vi "Get NextGen XML DataType For Control.vi"(8 "error in (no error)":errorcluster, 11 "Ctl Refnum":refnum<vi>) -> (0 "error out":errorcluster, 3 "String":string)   [LabVIEW 2020, in "Web Service Description.lvlib" / "NextGenXMLTypeGenerator.lvclass"]
uses:
  <vilib>/AppBuilder/Engine/WebServiceDescription/NextGenXMLTypeGenerator/NextGenXMLTypeGenerator.lvclass
  e:/builds/penguin/labview/branches/2020/dev/dist/vi.lib/AppBuilder/Engine/WebServiceDescription/LVDataTypes/LVTypeVisitor/LVTypeVisitor.lvclass
  <vilib>/AppBuilder/Engine/WebServiceDescription/LVDataTypes/LVType/LVType.lvclass
  <vilib>/AppBuilder/Engine/WebServiceDescription/LVDataTypes/LVDataTypes.lvlib
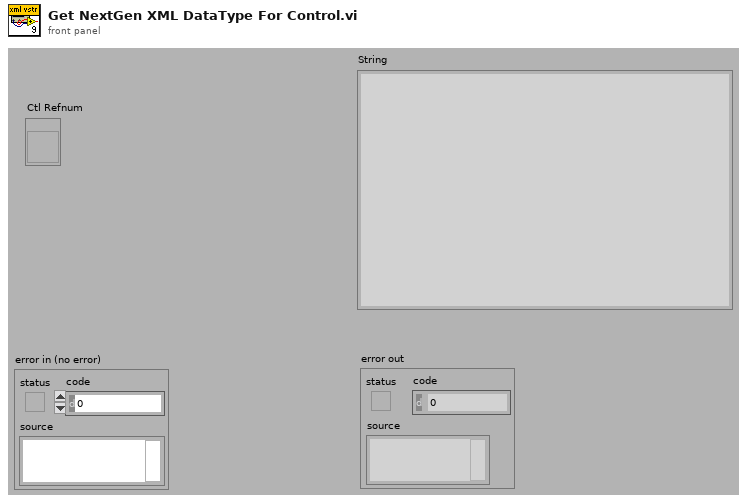
[diagram p1: front panel]
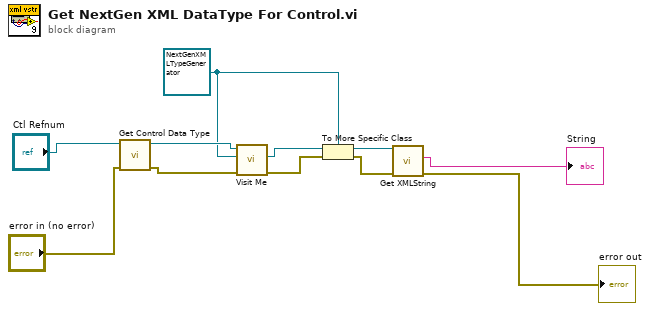
[diagram p0: block diagram]
diagram:
  w6 = refnum<class "NextGenXMLTypeGenerator.lvclass"> refnum ("NextGenXMLTypeGenerator.lvclass")
  n1 = call <vilib>:"Get Control Data Type.vi"("error in (no error)"="error in (no error)", "Ctl Refnum"="Ctl Refnum") -> ("error out"=w9:errorcluster, "Type"=w10:refnum<class "LVType.lvclass">)  [unwired: 8 out]
  n2 = call-dynamic "Visit Me.vi"("error in (no error)"=w9, "Visitor In"=w6, "LVType in"=w10) -> ("error out"=w8:errorcluster, "Visitor Out"=w7:refnum<class "LVTypeVisitor.lvclass">)  [unwired: 7 out]
  n3 = To More Specific Class(target class=w6, reference=w7, error in=w8) -> (specific class reference=w4:refnum<class "NextGenXMLTypeGenerator.lvclass">, error out=w5:errorcluster)
  n4 = call <vilib>:"Get XMLString.vi"("error in (no error)"=w5, "NextGenXMLTypeGenerator.lvclass in"=w4) -> ("error out"=→"error out":errorcluster, "XMLString"=→"String":string)  [unwired: 8 out]
